vi "Teleop.vi"(10 "Match Info":T2={"Autonomous Elapsed Seconds"=0.0, "TeleOp Elapsed Seconds"=0.0, "Disabled Elapsed Seconds"=0.0, "Visited Autonomous"=FALSE, "Visited TeleOp"=FALSE, "Visited Disabled"=FALSE, "Autonomous Settings"={"Autonomous Style"=enum."Independent", "VI Refnum"=refnum}}, 11 "Call Context":T3) -> ()   [LabVIEW 2017]
doc: "This VI is called for each enabled TeleOp packet received from the DS. It is typically used to read from joysticks and other inputs and update I/O or setpoints for timed control loops. It should complete and return within 20 milliseconds or risk missing DS packets."
uses:
  <vilib>/Rock Robotics/WPI/DriverStation/WPI_DriverStationDerivedRobotMode.ctl
  <vilib>/Rock Robotics/WPI/DriverStation/WPI_DriverStationMatch Info.ctl
  Typedef/XBox Axis.ctl
  Typedef/XBox Buttons.ctl
  <vilib>/Rock Robotics/WPI/Utilities/WPI_GetSetVariantRefNum.vi
  <vilib>/Rock Robotics/Network Tables/NT Write Boolean Array.vi
  <vilib>/Rock Robotics/Network Tables/NT Write Numeric Array.vi
  Elevator/Implementation/Elevator Position Global.vi
panel:
  in  "PIDF gains High Gear":T1
  in  "PIDF gains Low Gear":T1
  in  "Elevator Toggle Range":dbl=0.2
  in  "Elevator Speed":dbl=0.9 format="%#_13g"
  in  "QuesoTurn Sensitivty":dbl=0.7
  in  "Elevato PickUp Setpoint":dbl=10.0
  in  "Elevator Up Setpoint":dbl=45.0
  in  "Cheesy Sensitivity":dbl(slide)=0.7593984962406015 scale=0.0..1.0
  in  "Arcade to Queso":bool=TRUE
  # "<-- This is not motor speed!"
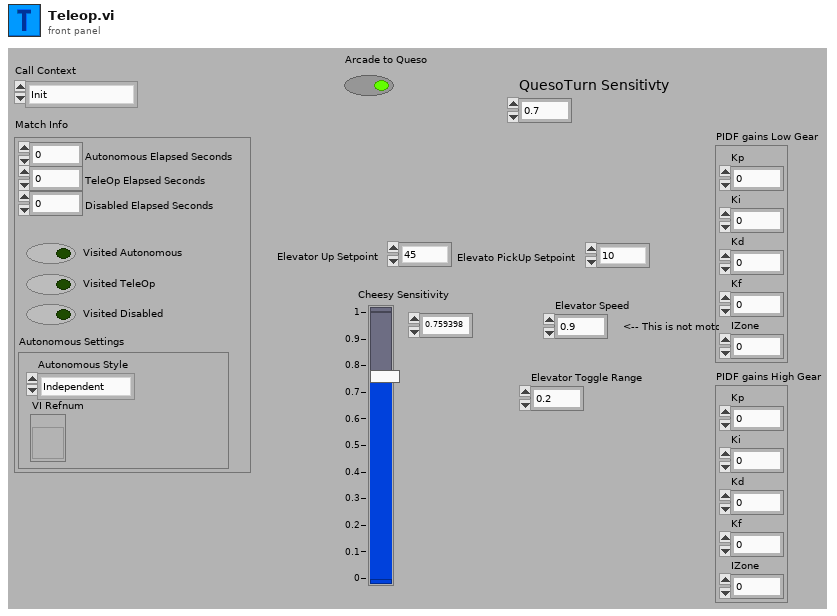
[diagram p1: front panel]
types:
  T1 = cluster{"Kp":dbl, "Ki":dbl, "Kd":dbl, "Kf":dbl, "IZone":dbl}
  T2 = typedef "WPI_DriverStationMatch Info.ctl" = cluster{"Autonomous Elapsed Seconds":dbl, "TeleOp Elapsed Seconds":dbl, "Disabled Elapsed Seconds":dbl, "Visited Autonomous":bool, "Visited TeleOp":bool, "Visited Disabled":bool, "Autonomous Settings":cluster{"Autonomous Style":enum16{"Iterative", "Independent"}, "VI Refnum":refnum<vi>}}
  T3 = typedef "WPI_DriverStationDerivedRobotMode.ctl" = enum16{"Init", "Execute", "Stop"}
  T4 = typedef "XBox Buttons.ctl" = enum16{"A", "B", "X", "Y", "Left Bumper", "Right Bumper", "Back", "Start", "Left Joystick", "Right Joystick"}
  T5 = typedef "XBox Axis.ctl" = enum16{"Left X", "Left Y", "Left Trigger", "Right Trigger", "Right X", "Right Y"}
  T6 = typedef "WPI_JoystickDevRef.ctl" = cluster{"Device":T7}
  T7 = typedef "WPI_JoystickDeviceEnum.ctl" = enum16{"USB 0", "USB 1", "USB 2", "USB 3", "USB 4", "USB 5"}
  T8 = typedef "TalonSRX6Motor.ctl" = cluster{"FrontLeftMaster":T9, "FrontLeftSlave1":T9, "FrontLeftSlave2":T9, "FrontRightMaster":T9, "FrontRightSlave1":T9, "FrontRightSlave2":T9}
  T9 = typedef "WPI_MotorControlDeviceRef.ctl" = cluster{"DeviceStatus":errorcluster, "Type":T10, "PWM":cluster{"PWM Channel":T11, "DeadBand":T12}, "CAN":cluster{"Device Number":u8, "SetOutput VI Ref":variant, "GetOutput VI Ref":variant, "Enable VI Ref":variant, "Disable VI Ref":variant, "Data":variant}, "Invert":bool, "DIO PWM":cluster{"PWM \"Enable\" Channel":T11, "DIOChannel":T13, "PWM Rate":dbl}}
  T10 = typedef "WPI_MotorControlType.ctl" = enum16{"PWM", "CAN", "DIO PWM"}
  T11 = typedef "FPGA_DIOPWMChannel.ctl" = enum8{"PWM 0", "PWM 1", "PWM 2", "PWM 3", "PWM 4", "PWM 5", "PWM 6", "PWM 7", "PWM 8", "PWM 9", "PWM MXP 0", "PWM MXP 1", "PWM MXP 2", "PWM MXP 3", "PWM MXP 4", "PWM MXP 5", "PWM MXP 6", "PWM MXP 7", "PWM MXP 8", "PWM MXP 9", "Invalid"}
  T12 = typedef "WPI_PWMDeadband.ctl" = cluster{"Name":string, "maxPositivePwm":i32, "minPositivePwm":i32, "centerPwm":i32, "maxNegativePwm":i32, "minNegativePwm":i32, "angularRange":u16}
  T13 = typedef "FPGA_DIOChannel.ctl" = enum8{"DIO 0", "DIO 1", "DIO 2", "DIO 3", "DIO 4", "DIO 5", "DIO 6", "DIO 7", "DIO 8", "DIO 9", "DIO MXP 0", "DIO MXP 1", "DIO MXP 2", "DIO MXP 3", "DIO MXP 4", "DIO MXP 5", "DIO MXP 6", "DIO MXP 7", "DIO MXP 8", "DIO MXP 9", "DIO MXP 10", "DIO MXP 11", "DIO MXP 12", "DIO MXP 13", "DIO MXP 14", "DIO MXP 15", "SPI Port CS1", "SPI Port CS2", "SPI Port CS3", "SPI Port MISO", "SPI Port MOSI", "Invalid"}
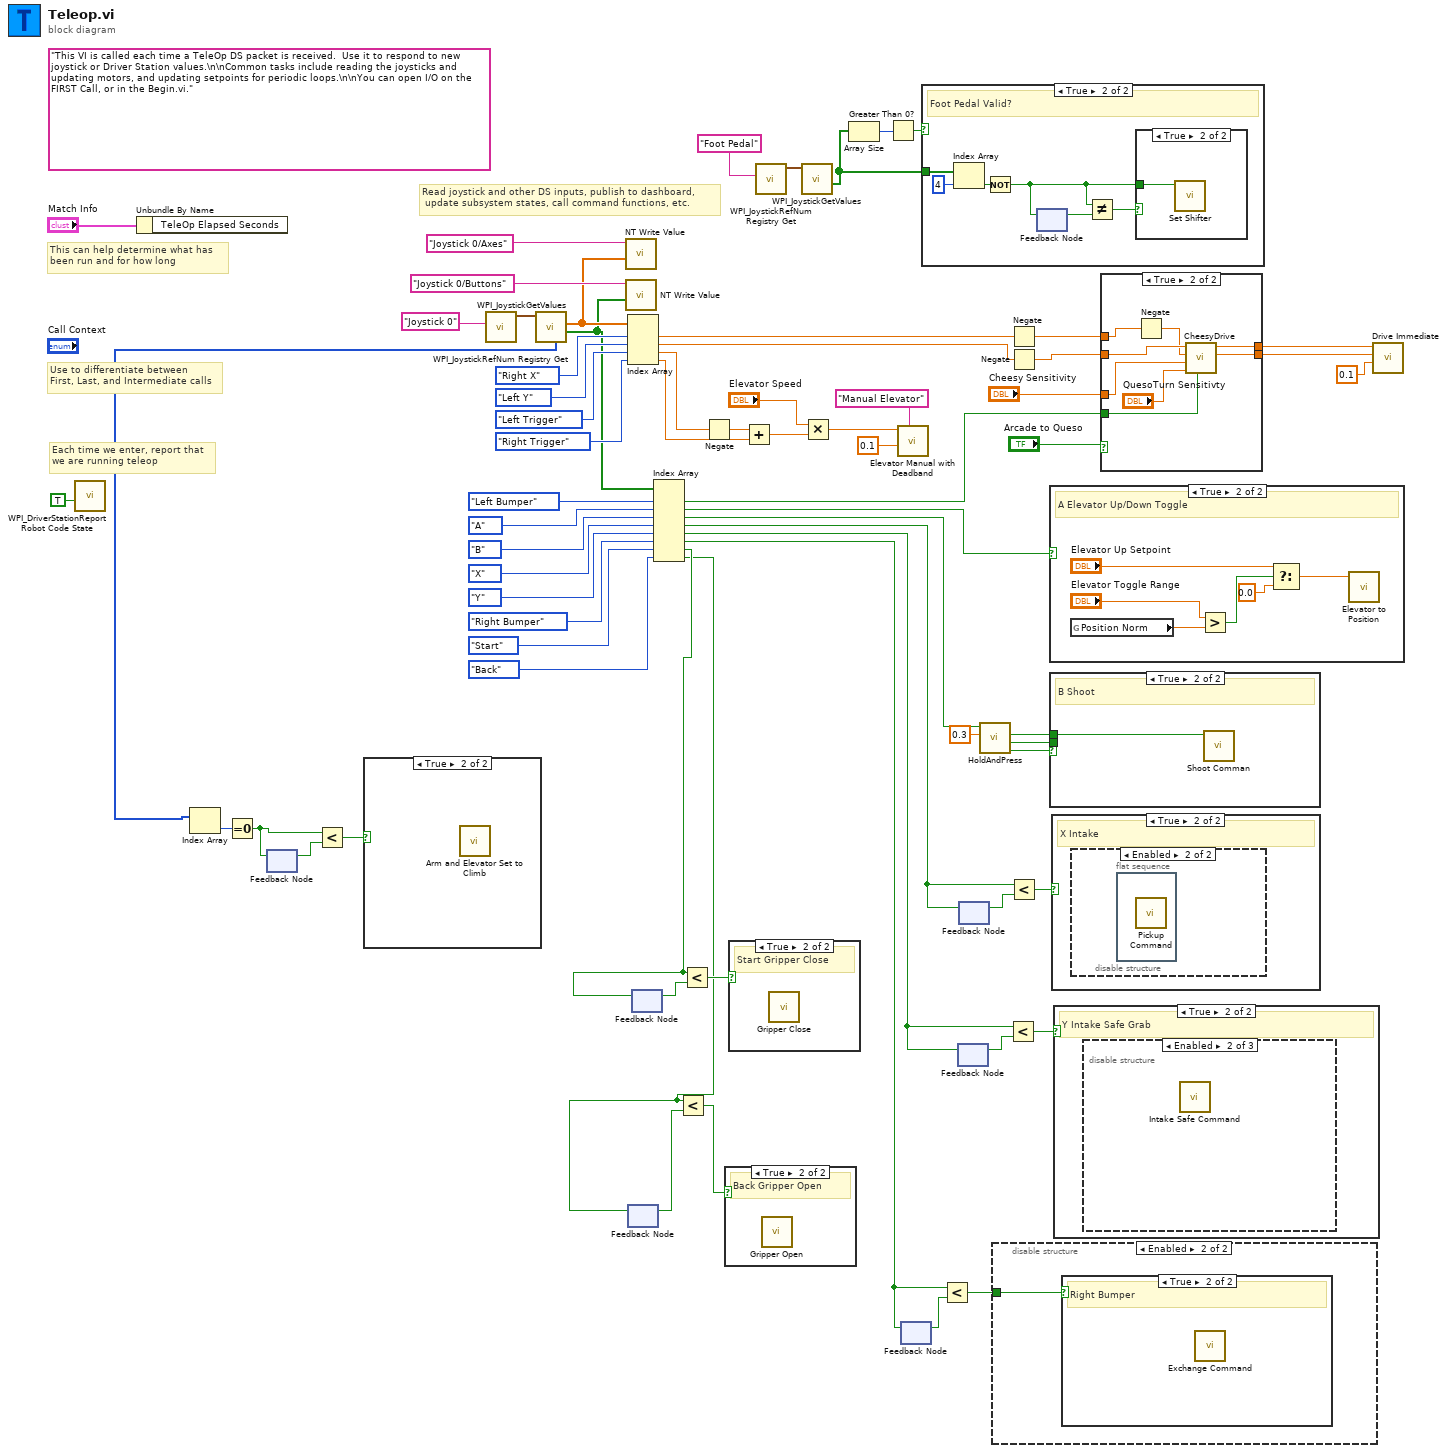
[diagram p0: block diagram]
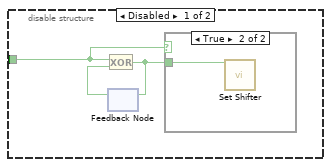
[diagram p3: hidden frame]
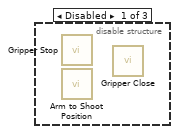
[diagram p12: hidden frame]
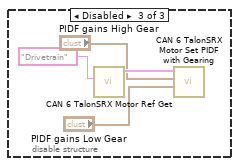
[diagram p13: hidden frame]
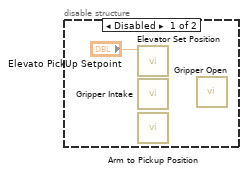
[diagram p15: hidden frame]
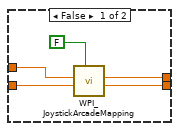
[diagram p17: hidden frame]
diagram:
  (unwired) "This VI is called each time a TeleOp DS packet is received.  Use it to respond to new joystick or Driver Station values.\n\nCommon tasks include reading the joysticks and updating motors, and updating setpoints for periodic loops.\n\nYou can open I/O on the FIRST Call, or in the Begin.vi."
  # "Read joystick and other DS inputs, publish to dashboard,\n update subsystem states, call command functions, etc."
  # "Each time we enter, report that\nwe are running teleop"
  # "Use to differentiate between\nFirst, Last, and Intermediate calls"
  # "This can help determine what has\nbeen run and for how long"
  n1 = call <vilib>:"WPI_DriverStationReport Robot Code State.vi"("TeleOp"=TRUE ("Autonomous")) -> ()  [unwired: 10 in, 1 out]
  n2 = Unbundle By Name("Match Info") -> ()  [unwired: 1 out]
  n3 = feedback #1() -> (w5:bool)  [unwired: 1 in]
  n4 = call <vilib>:"WPI_JoystickRefNum Registry Get.vi"("refnum name"="Joystick 0") -> ("JoystickDevRef"=w66:T6)  [unwired: 1 in, 9 out]
  n5 = call <vilib>:"WPI_JoystickGetValues.vi"("JoystickDevRef"=w66) -> ("Buttons"=w32:bool[], "Axes"=w63:dbl[], "POVs"=w3:i16[])  [unwired: 6 in, 2 out]
  n6 = Index Array(array=w3) -> (element=w2:i16)  [unwired: 1 in]
  n7 = Equal To 0?(x=w2) -> (x = 0?=w1:bool)
  n8 = feedback-in #1(w1) -> ()
  n9 = Less?(x=w1, y=w5) -> (x < y?=w4:bool)
  n10 = case shown="True" w4 {
    frame False {
    }
    frame True {
      n11 = call "Arm and Elevator Set to Climb.vi"() -> ()  [unwired: 11 in, 1 out]
    }
  }
  n12 = call-poly <vilib>:"NT Write Value.vi"("Numeric Array"=w63, "Name"="Joystick 0/Axes") -> ()  [unwired: 9 in, 1 out]
  n13 = call-poly <vilib>:"NT Write Value.vi"("Boolean Array"=w32, "Name"="Joystick 0/Buttons") -> ()  [unwired: 9 in, 1 out]
  n14 = Index Array(array=w63, index #1=XBox_Axis."Right X" ("Enum"), index #2=XBox_Axis."Left Y" ("Enum"), index #3=XBox_Axis."Left Trigger" ("Enum"), index #4=XBox_Axis."Right Trigger" ("Enum")) -> (element #1=w59:dbl, element #2=w65:dbl, element #3=w43:dbl, element #4=w42:dbl)
  n15 = feedback #2() -> (w22:bool)  [unwired: 1 in]
  n16 = feedback #3() -> (w26:bool)  [unwired: 1 in]
  n17 = Index Array(array=w32, index #1=XBox_Buttons."Left Bumper" ("Enum"), index #2=XBox_Buttons."A" ("Enum"), index #3=XBox_Buttons."B" ("Enum"), index #4=XBox_Buttons."X" ("Enum"), index #5=XBox_Buttons."Y" ("Enum"), index #6=XBox_Buttons."Right Bumper" ("Enum"), index #7=XBox_Buttons."Start" ("Enum"), index #8=XBox_Buttons."Back" ("Enum")) -> (element #1=w11:bool, element #2=w46:bool, element #3=w10:bool, element #4=w38:bool, element #5=w35:bool, element #6=w30:bool, element #7=w24:bool, element #8=w21:bool)
  n18 = feedback-in #2(w21) -> ()
  n19 = feedback-in #3(w24) -> ()
  n20 = Less?(x=w21, y=w22) -> (x < y?=w23:bool)
  n21 = Less?(x=w24, y=w26) -> (x < y?=w25:bool)
  n22 = Negate(x=w43) -> (-x=w34:dbl)
  n23 = case shown="True" w23 {
    frame False {
    }
    frame True {
      # "Back Gripper Open"
      n24 = call "Gripper Open.vi"() -> ()  [unwired: 11 in, 1 out]
    }
  }
  n25 = case shown="True" w25 {
    frame False {
    }
    frame True {
      # "Start Gripper Close"
      n26 = call "Gripper Close.vi"() -> ()  [unwired: 11 in, 1 out]
    }
  }
  n27 = Add(x=w34, y=w42) -> (x+y=w41:dbl)
  n28 = call <vilib>:"WPI_JoystickRefNum Registry Get.vi"("refnum name"="Foot Pedal") -> ("JoystickDevRef"=w19:T6)  [unwired: 9 in, 1 out]
  n29 = call <vilib>:"WPI_JoystickGetValues.vi"("JoystickDevRef"=w19) -> ("Buttons"=w17:bool[])  [unwired: 6 in, 4 out]
  n30 = Multiply(x="Elevator Speed", y=w41) -> (x*y=w14:dbl)
  n31 = Array Size(array=w17) -> (size(s)=w18:i32)
  n32 = Greater Than 0?(x=w18) -> (x > 0?=w16:bool)
  n33 = call "Elevator Manual with Deadband.vi"("Description"="Manual Elevator", "Deadband Value"=0.1, "Setpoint"=w14) -> ()  [unwired: 8 in, 1 out]
  n34 = feedback-in #4(w30) -> ()
  n35 = feedback #4() -> (w31:bool)  [unwired: 1 in]
  n36 = case shown="True" w16 {
    tunnel: w17 -> [_ w73]
    frame False {
    }
    frame True {
      # "Foot Pedal Valid?"
      n37 = Index Array(array=w73, index=4) -> (element=w71:bool)
      n38 = Not(x=w71) -> (.not. x?=w70:bool)
      n39 = feedback #5() -> (w75:bool)  [unwired: 1 in]
      n40 = feedback-in #5(w70) -> ()
      n41 = Not Equal?(x=w70, y=w75) -> (x != y?=w74:bool)
      n42 = case shown="True" w74 {
        tunnel: w70 -> [_ w76]
        frame False {
        }
        frame True {
          n43 = call "Set Shifter.vi"("High Gear?"=w76) -> ()  [unwired: 10 in, 1 out]
        }
      }
    }
  }
  n44 = Less?(x=w30, y=w31) -> (x < y?=w29:bool)
  n45 = feedback #6() -> (w37:bool)  [unwired: 1 in]
  n46 = feedback-in #6(w35) -> ()
  n47 = feedback-in #7(w38) -> ()
  n48 = feedback #7() -> (w39:bool)  [unwired: 1 in]
  n49 = call "HoldAndPress.vi"("Holdtime"=0.3, "Input"=w10) -> ("Press?"=w8:bool, "Long Press"=w6:bool, "Quick Press"=w7:bool)  [unwired: 4 in, 3 out]
  n50 = disable-structure shown="Enabled" {
    disable-tunnel: w29 -> [w77 w81]
    frame Disabled {
      n51 = feedback #8() -> (w79:bool)  [unwired: 1 in]
      n52 = Exclusive Or(1:w79, 2:w77) -> (0:w78:bool)
      n53 = feedback-in #8(w78) -> ()
      n54 = case shown="True" w77 {
        tunnel: w78 -> [_ w80]
        frame False {
        }
        frame True {
          n55 = call "Set Shifter.vi"("High Gear?"=w80) -> ()  [unwired: 10 in, 1 out]
        }
      }
    }
    frame Enabled {
      n56 = case shown="True" w81 {
        frame False {
        }
        frame True {
          # "Right Bumper"
          n57 = call "Exchange Command.vi"() -> ()  [unwired: 11 in, 1 out]
        }
      }
    }
  }
  n58 = Less?(x=w35, y=w37) -> (x < y?=w36:bool)
  n59 = Negate(x=w59) -> (-x=w57:dbl)
  n60 = Negate(x=w65) -> (-x=w58:dbl)
  n61 = Less?(x=w38, y=w39) -> (x < y?=w40:bool)
  n62 = case shown="True" w46 {
    frame False {
    }
    frame True {
      # "A Elevator Up/Down Toggle"
      n63 = global read "Elevator Position Global.vi" "Position Norm"() -> (w87:dbl)
      n64 = Greater?(x="Elevator Toggle Range", y=w87) -> (0:w85:bool)
      n65 = Select(t="Elevator Up Setpoint", s=w85, f=0.0) -> (s? t:f=w84:dbl)
      n66 = call "Elevator to Position.vi"("Value"=w84) -> ()  [unwired: 10 in, 1 out]
    }
  }
  n67 = case shown="True" w8 {
    tunnel: w7 -> [_ w88]
    tunnel: w6 -> [_ _]
    frame False {
    }
    frame True {
      # "B Shoot"
      n68 = call "Shoot Comman.vi"("Soft Shot?"=w88) -> ()  [unwired: 10 in, 1 out]
    }
  }
  n69 = case shown="True" w40 {
    frame False {
    }
    frame True {
      # "X Intake"
      n70 = disable-structure shown="Enabled" {
        frame Disabled {
          n71 = call "Elevator Set Position.vi"("Setpoint"="Elevato PickUp Setpoint") -> ()  [unwired: 10 in, 1 out]
          n72 = call "Gripper Intake.vi"() -> ()  [unwired: 11 in, 1 out]
          n73 = call "Arm to Pickup Position.vi"() -> ()  [unwired: 11 in, 1 out]
          n74 = call "Gripper Open.vi"() -> ()  [unwired: 11 in, 1 out]
        }
        frame Enabled {
          n75 = flat-sequence {
            frame #0 {
              n76 = call "Pickup Command.vi"() -> ()  [unwired: 11 in, 1 out]
            }
          }
        }
      }
    }
  }
  n77 = case shown="True" w36 {
    frame False {
    }
    frame True {
      # "Y Intake Safe Grab"
      n78 = disable-structure shown="Enabled" {
        frame Disabled {
          n79 = call "Gripper Stop.vi"() -> ()  [unwired: 11 in, 1 out]
          n80 = call "Arm to Shoot Position.vi"() -> ()  [unwired: 11 in, 1 out]
          n81 = call "Gripper Close.vi"() -> ()  [unwired: 11 in, 1 out]
        }
        frame Enabled {
          n82 = call "Intake Safe Command.vi"() -> ()  [unwired: 11 in, 1 out]
        }
        frame Disabled {
          n83 = call "CAN 6 TalonSRX Motor Ref Get.vi"("refnum name"="Drivetrain") -> ("TalonSRX6MotorRef out"=w92:T8)  [unwired: 9 in, 1 out]
          n84 = call "CAN 6 TalonSRX Motor Set PIDF with Gearing.vi"("PIDF gains Low Gear"="PIDF gains Low Gear", "PIDF gains High Gear"="PIDF gains High Gear", "TalonSRX6MotorRef"=w92) -> ()  [unwired: 8 in, 1 out]
        }
      }
    }
  }
  n85 = case shown="True" "Arcade to Queso" {
    tunnel: w58 -> [w97 w103]
    tunnel: w57 -> [w98 w102]
    tunnel: [w96 w106] -> w55
    tunnel: [w95 w105] -> w54
    tunnel: w11 -> [_ w104]
    tunnel: "Cheesy Sensitivity" -> [_ w100]
    frame False {
      n86 = call <vilib>:"WPI_JoystickArcadeMapping.vi"("Square Inputs"=FALSE, "Y axis value"=w97, "X axis value"=w98) -> ("Right Motor Value"=w96:dbl, "Left Motor Value"=w95:dbl)  [unwired: 7 in]
    }
    frame True {
      n87 = Negate(x=w102) -> (-x=w101:dbl)
      n88 = call "CheesyDrive.vi"("Quickturn"=w104, "QuickTurn Sensitivty"="QuesoTurn Sensitivty", "Sensitivty"=w100, "Wheel"=w101, "Throttle"=w103) -> ("Right PWM"=w106:dbl, "Left PWM"=w105:dbl)  [unwired: 5 in]
    }
  }
  n89 = call "Drive Immediate.vi"("Deadband Value"=0.1, "Right Setpoint"=w55, "Left Setpoint"=w54) -> ()  [unwired: 8 in, 1 out]
